vi "Rohde_TurnOff_PS.vi"() -> ()   [LabVIEW 2018]
panel:
  out "error out":errorcluster
  in  "error in (no error)":errorcluster
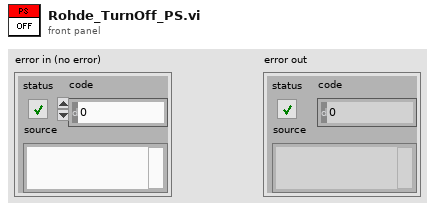
[diagram p1: front panel]
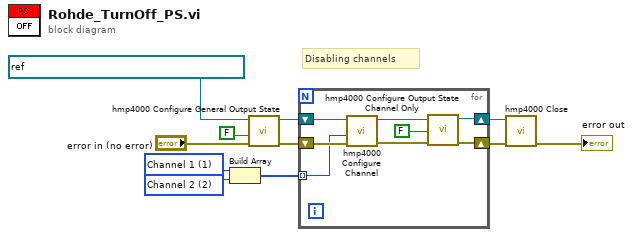
[diagram p0: block diagram]
diagram:
  w11 = 2 items=["Channel 1"=1, "Channel 2"=2, "Channel 3"=3, "Channel 4"=4] ("Channel (Channel 1)")
  w10 = 1 items=["Channel 1"=1, "Channel 2"=2, "Channel 3"=3, "Channel 4"=4] ("Channel (Channel 1)")
  # "Disabling channels"
  n1 = Build Array(w10, w11) -> (w7:i32[])
  n2 = call "hmp4000 Configure General Output State.vi"("error in (no error)"="error in (no error)", "Output State (Off)"=FALSE, "VISA resource name"=refnum<visa-resource-name> "TCPIP::10.42.0.201::5025::SOCKET") -> ("error out"=w5:errorcluster, "VISA resource name out"=w4:refnum<visa-resource-name>)  [unwired: 7 in]
  n3 = for {
    tunnel: w7 -> [w17] mode=indexing
    shift-right: [w13] -> w9
    shift-left: w5 -> [w19]
    shift-right: [w12] -> w8
    shift-left: w4 -> [w18]
    n4 = call "hmp4000 Configure Channel.vi"("error in (no error)"=w19, "Channel (Channel 1)"=w17, "VISA resource name"=w18) -> ("error out"=w15:errorcluster, "VISA resource name out"=w14:refnum<visa-resource-name>)  [unwired: 7 in]
    n5 = call "hmp4000 Configure Output State Channel Only.vi"("error in (no error)"=w15, "Output State (Off)"=FALSE ("t"), "VISA resource name"=w14) -> ("error out"=w13:errorcluster, "VISA resource name out"=w12:refnum<visa-resource-name>)  [unwired: 7 in]
  }
  n6 = call "hmp4000 Close.vi"("error in (no error)"=w9, "VISA resource name"=w8) -> ("error out"=→"error out":errorcluster)  [unwired: 9 in]
